vi "PS35_MoveEx.vi"(0 "Control unit ID":i32=1 min=1 max=10, 5 "Axis number":i32=1 min=1 max=3, 7 "dValue":dbl step=0.01 format="%.4f", 9 "nEx":i32 min=0 max=1, 11 "error in (no error)":errorcluster) -> (15 "error out":errorcluster)   [LabVIEW 2020]
doc: "PS35_MoveEx.vi, created: 06.03.2009 alex; last change: 22.10.2019 alex;\n\n<B>FUNCTION:</B> \n\nDrive an axis to a new target position or a distance.\nAt first a new target position of an axis is defined. Then an axis goes to a new\ntarget position or a distance either in the trapezoidal or S-curve profile. This is\nvalid only for released axes.\n----------------------------------------------------------------------------------------\n<B>INPUT:</B>\n[I32] <B>Control unit ID:</B> control unit index. (Default=1, Range=1...10) \n[I32] <B>Axis number:</B> axis number. (Default=1, Range=1...3) \n[DBL] <B>dValue:</B> new target position. (Default=0.0) \n[I32] <B>nEx:</B> define values of the target position. (Default=0, Range=0...1)\n0 - new target position (values in increments),\n1 - new target position (values in selected unit). \n[CLU] <B>error in</B>\n----------------------------------------------------------------------------------------\n<B>OUTPUT:</B>\n[CLU] <B>error out</B>\n----------------------------------------------------------------------------------------\n<B>SUB-VIs:</B>\n----------------------------------------------------------------------------------------\n<B>EXT-Calls:</B>\nps35.dll (V2.01)\n----------------------------------------------------------------------------------------"
uses:
  ps35.dll
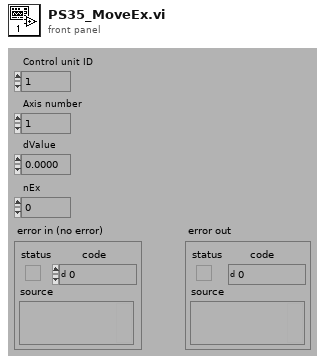
[diagram p1: front panel]
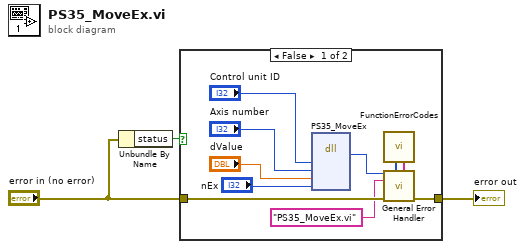
[diagram p0: block diagram]
diagram:
  n1 = Unbundle By Name("error in (no error)") -> ("status"=w1:bool)
  n2 = case shown="False" w1 {
    tunnel: "error in (no error)" -> [w12 w14]
    tunnel: [w11 w14] -> w3
    frame False {
      n3 = dll-call lib="C:/GEECS/Developers Version/source/Device Drivers/OwiSoft_PS35/OWISoftOEM/ps35/labview/lv82/ps35.dll" fn="PS35_MoveEx" label="PS35_\nMoveEx"("Index"="Control unit ID", "AxisNr"="Axis number", "dValue"="dValue", "nEx"="nEx") -> ("Rückgabetyp"=w10:i32)  [unwired: 7 in, 2 out]
      n4 = call "FunctionErrorCodes.vi"() -> ("[user-defined codes]"=w5:i32[], "[user-defined descriptions]"=w4:string[])  [unwired: 8 in]
      n5 = call "General Error Handler.vi"("[error code] (0)"=w10, "[user-defined codes]"=w5, "[user-defined descriptions]"=w4, "[error source] (\" \")"="PS35_MoveEx.vi" ("[error source] (\" \")"), "error in (no error)"=w12) -> ("error out"=w11:errorcluster)  [unwired: 6 in, 4 out]
    }
    frame True {
    }
  }
  "error out" <- w3
